vi "Request Task Setpoint.vi"(7 "Task Ident":string, 8 "error in":errorcluster, 10 "Setpoint Ident":string, 11 "ISeries Actor in":refnum<class "ISeries Actor.lvclass">) -> (0 "error out":errorcluster, 3 "ISeries Actor out":refnum<class "ISeries Actor.lvclass">)   [LabVIEW 2024, in "ISeries Actor.lvlib" / "ISeries Actor.lvclass"]
uses:
  ISeries Actor.lvclass
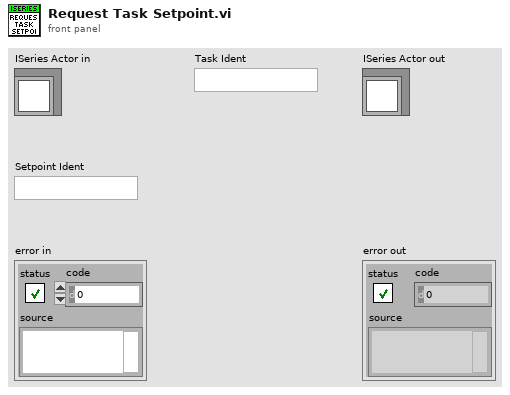
[diagram p1: front panel]
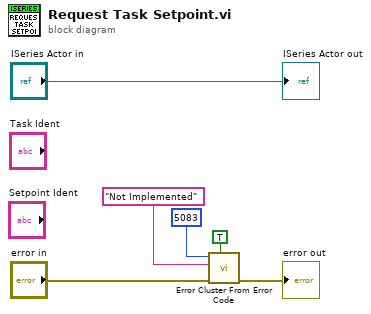
[diagram p0: block diagram]
diagram:
  n1 = call <vilib>:"Error Cluster From Error Code.vi"("show call chain? (False)"=TRUE, "error in (no error)"="error in", "error message (\"\")"="Not Implemented" ("error message (\"\")"), "error code (0)"=5083) -> ("error out"=→"error out":errorcluster)  [unwired: 5 in]
  "ISeries Actor out" <- "ISeries Actor in"
